vi "Create Response.vi"(6 "id":string, 8 "error in (no error)":errorcluster, 10 "result":variant, 11 "JSON-RPC in":refnum<class "JSON-RPC.lvclass">) -> (0 "error out":errorcluster, 2 "{JSON} Response":string, 3 "JSON-RPC out":refnum<class "JSON-RPC.lvclass">)   [LabVIEW 2019, in "JSON-RPC.lvclass"]
uses:
  JSON-RPC.lvclass
  private/Create Response-JSONtext.vi/31d5db40-9dcb-43d1-a6f6-9a2e0a5d4432.vi
  private/Create Response-JSONtext.vi/c6edfa98-d038-4790-952c-164baa6befaa.vi
  private/Create Response-JSONtext.vi/8b9e59fa-9ebd-4504-a939-6047597c77d3.vi
  private/Create Error Object.vi
  <vilib>/JDP Science/JSONtext/Variant to JSON Text.vi
  <vilib>/JDP Science/JSONtext/Set Item.vi
  <vilib>/JDP Science/JSONtext/LVClass Serializer/JSONtext LVClass Serializer.lvclass
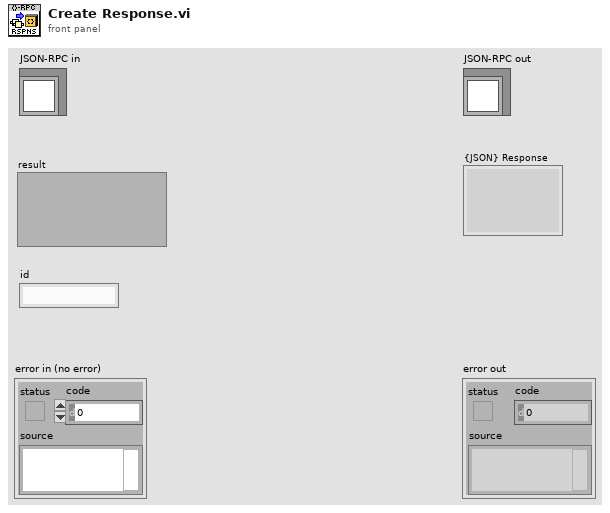
[diagram p1: front panel]
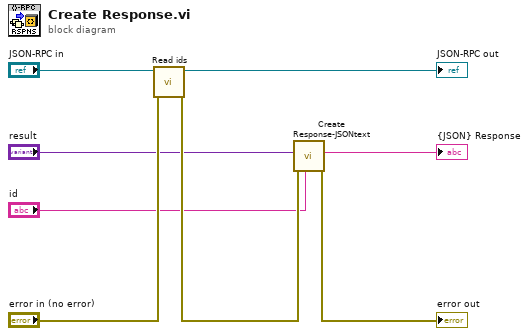
[diagram p0: block diagram]
diagram:
  n1 = call "Read ids.vi"("error in (no error)"="error in (no error)", "JSON-RPC in"="JSON-RPC in") -> ("error out"=w5:errorcluster, "JSON-RPC out"=→"JSON-RPC out":refnum<class "JSON-RPC.lvclass">)  [unwired: 7 in, 1 out]
  n2 = call "Create Response-JSONtext.vi"("id"="id", "error in (no error)"=w5, "result"="result") -> ("error out"=→"error out":errorcluster, "{JSON}"=→"{JSON} Response":string)  [unwired: 7 in]
